vi "Main.vi"() -> ()   [LabVIEW 2024]
doc: "This small application is only a proof of concept. When we have parameters or user data inside an application that could be modified (by the user) at run time, it is important that those changes are 'memorized' when the application is shut down. The next time the application is started it should keep the last configuration made. This is what this application does.\n\nEvery time the user changes the FP data, the changes are saved in the .ini file. If the user closes the application, the FP data is already saved in the .ini configuration file. The next time it is turned on, the data will be loaded again.\n\nIf the user modifies any tag or sector name, or any key name (or its value) in the configuration file (and saves these changes) at run time, the Update button updates this information in the FP of the application, it is the data of the gray fields. This may not be useful in a real application."
uses:
  controls/UI Data.ctl
  dependencies/config data path.ctl
  support/Message Queue/Enqueue Message (Array).vi
  support/Message Queue/Enqueue Message (Single).vi
  <vilib>/Utility/error.llb/Error Cluster From Error Code.vi
  <vilib>/ErrorRing/Error Ring.xnode
  support/Message Queue/Message Queue.lvlib
  support/User Event - Stop/User Event - Stop.lvlib
  dependencies/API Path Config Files Management.lvlib
panel:
  in  "folder path":path
  in  "xml file path":path
  out "Display value":string
  in  "Exit":bool
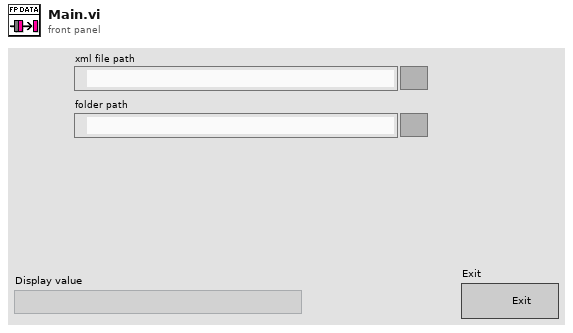
[diagram p1: front panel]
types:
  T1 = typedef "UI Data.ctl" = cluster{"Data Display Ref":refnum<vi>, "Exit Button Ref":refnum<vi>, "xml file Ref":refnum<vi>, "folder path Ref":refnum<vi>, "user path data":T2, "path value idx":i32[]}
  T2 = typedef "API Path Config Files Management.lvlib/config data path.ctl" = cluster{"sections":string[][], "key names":string[], "values":path[]}
  T3 = typedef "NI_LVConfig.lvlib/Config Data RefNum.ctl" = refnum<k1>
  T4 = typedef "Message Queue.lvlib/All Message Queues.ctl" = cluster{"UI":refnum<queue>}
  T5 = enum32{"existing file", "new file", "new or existing file", "existing dir", "new dir", "new or existing dir", "existing file (use LLBs)", "new file (use LLBs)", "new or existing file (use LLBs)", "new or existing file or directory (use LLBs)", "existing dir (use LLBs)", "new dir (use LLBs)", "new or existing dir (use LLBs)", "existing file or dir", "new file or dir", "new or existing file or dir", "existing file or dir (use LLBs)", "new file or dir (use LLBs)"}
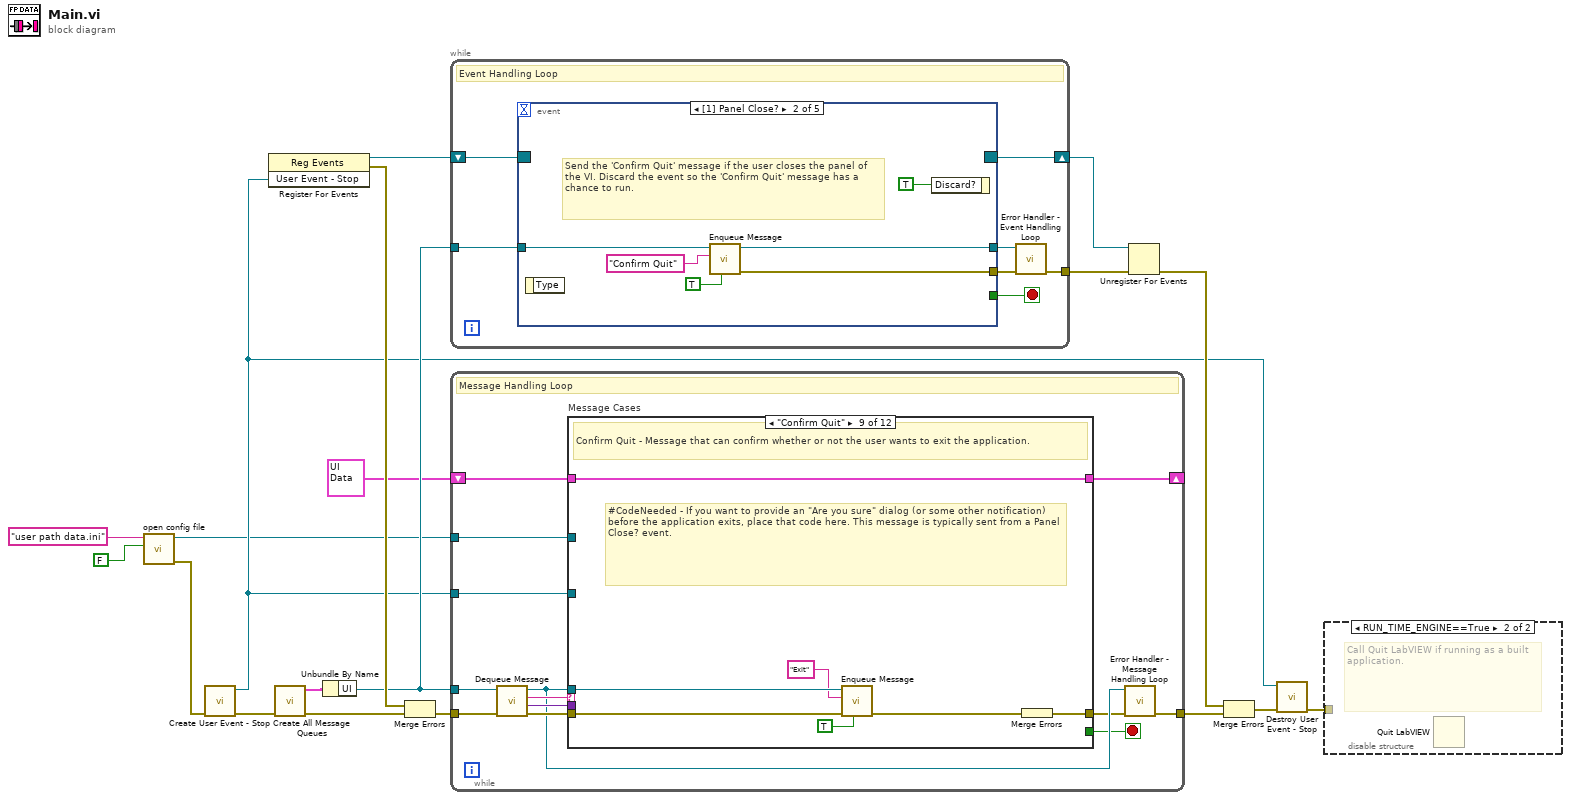
[diagram p0: block diagram]
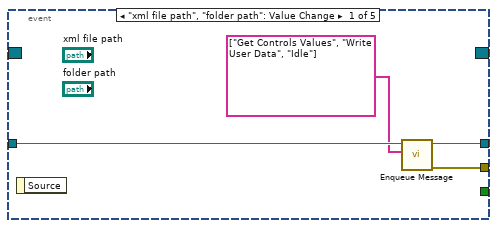
[diagram p3: hidden frame]
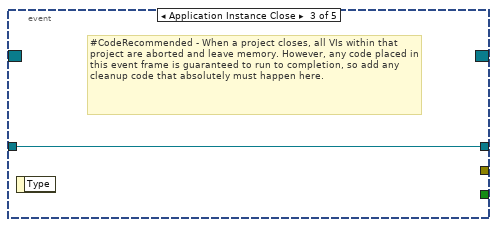
[diagram p4: hidden frame]
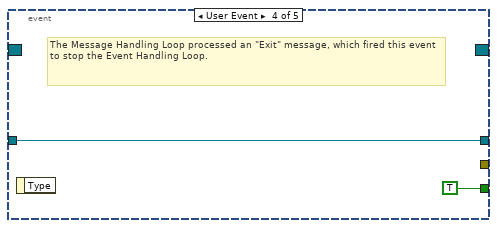
[diagram p5: hidden frame]
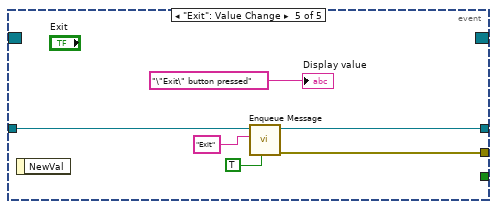
[diagram p6: hidden frame]
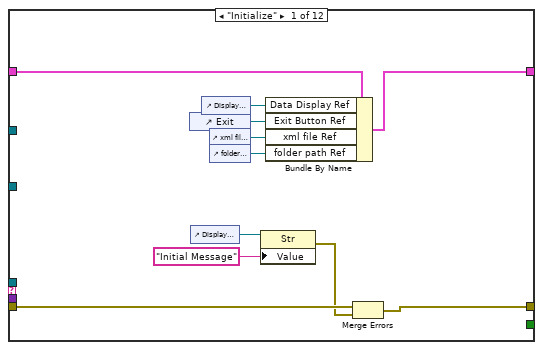
[diagram p7: hidden frame]
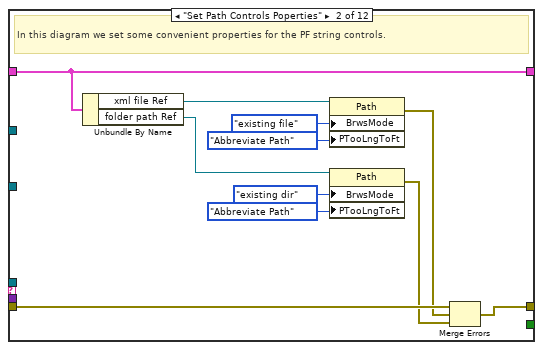
[diagram p8: hidden frame]
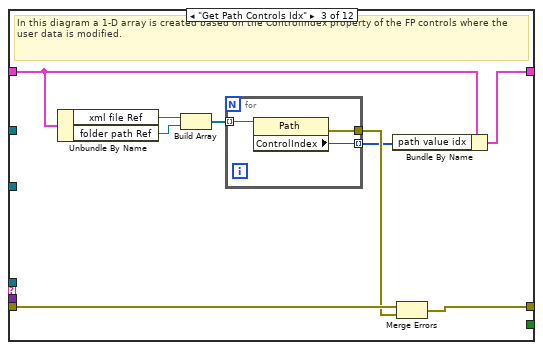
[diagram p9: hidden frame]
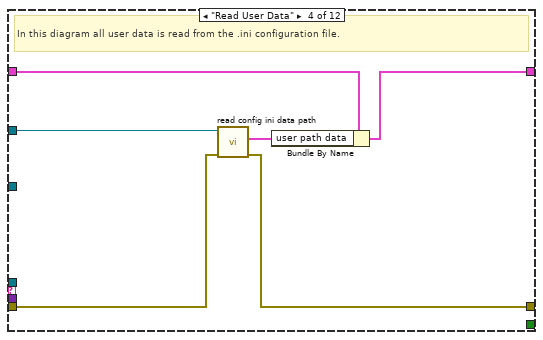
[diagram p10: hidden frame]
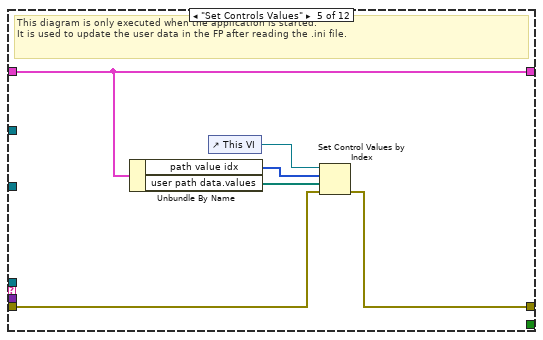
[diagram p11: hidden frame]
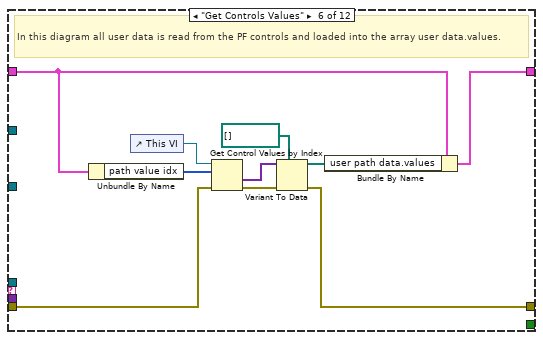
[diagram p12: hidden frame]
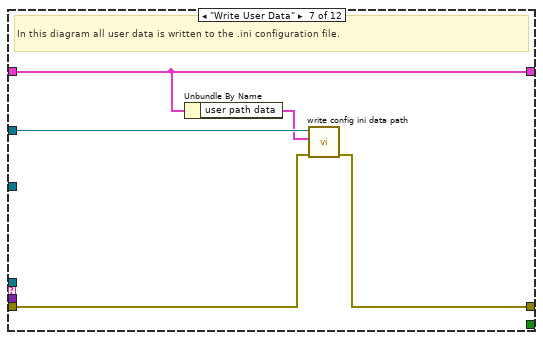
[diagram p13: hidden frame]
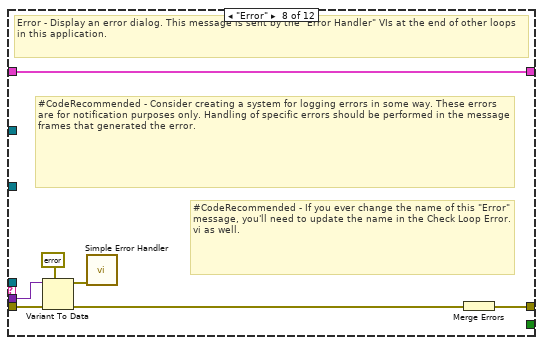
[diagram p14: hidden frame]
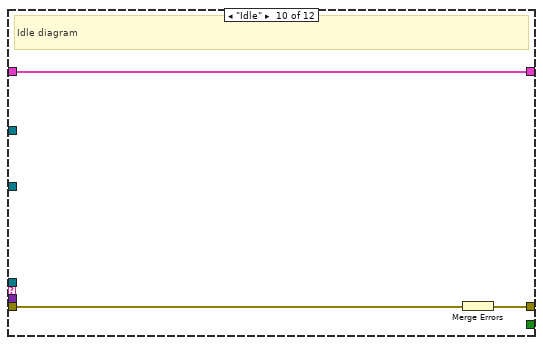
[diagram p15: hidden frame]
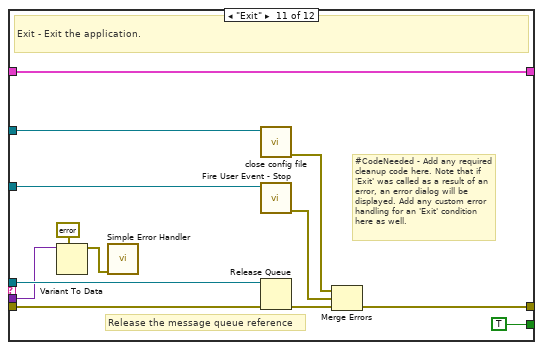
[diagram p16: hidden frame]
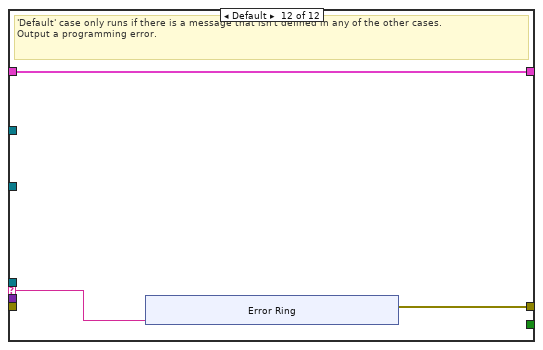
[diagram p17: hidden frame]
diagram:
  n1 = call "open config file.vi"("create file if necessary (T)"=FALSE, "file name"="user path data.ini") -> ("error out"=w2:errorcluster, "Refnum out"=w1:T3)  [unwired: 7 in, 1 out]
  n2 = call "Create User Event - Stop.vi"("error in (no error)"=w2) -> ("error out"=w14:errorcluster, "User Event - Stop"=w5:refnum<user-event>)  [unwired: 9 in]
  n3 = register-events(w5) -> (reference out=w7:refnum<event-registration>, error out=w19:errorcluster)  [unwired: 2 in]
  n4 = call "Create All Message Queues.vi"("error in (no error)"=w14) -> ("error out"=w18:errorcluster, "Message Queues out"=w17:T4)  [unwired: 9 in]
  n5 = Unbundle By Name(w17) -> ("UI"=w15:refnum<queue>)
  n6 = Merge Errors(w19, w18) -> (w6:errorcluster)
  n7 = while {
    tunnel: w15 -> [w26]
    shift-right: [w24] -> w11
    shift-left: w7 -> [w25]
    tunnel: [w20] -> w8
    stop <- w22 stop-if-true
    # "Event Handling Loop"
    n8 = event shown="[1] Panel Close?" {
      selector: w25 -> [_ _ _ _ _]
      dyn-events: [_ _ _ _ _] -> w24
      timeout: _ -> [_ _ _ _ _]
      tunnel: [_ _ _ TRUE ("Discard?") _] -> w22
      tunnel: w26 -> [w30 w35 w37 w39 w45]
      tunnel: [w28 w34 _ _ w44] -> w23
      tunnel: [w29 w33 w37 w39 w43] -> w21
      event "xml file path", "folder path": Value Change {
        n9 = event-data() -> ()  [unwired: 1 in, 1 out]
        n10 = call-poly "Enqueue Message.vi"("Message Array"=string[] ["Get Controls Values", "Write User Data", "Idle"], "Message Queue"=w30) -> ("error out"=w28:errorcluster, "dup Message Queue"=w29:refnum<queue>)  [unwired: 8 in]
      }
      event Panel Close? {
        # "Send the 'Confirm Quit' message if the user closes the panel of the VI. Discard the event so the 'Confirm Quit' message has a chance to run."
        n11 = event-data() -> ()  [unwired: 1 in, 1 out]
        n12 = call-poly "Enqueue Message.vi"("Priority Message? (F)"=TRUE, "Message"="Confirm Quit", "Message Queue"=w35) -> ("error out"=w34:errorcluster, "dup Message Queue"=w33:refnum<queue>)  [unwired: 7 in]
        n13 = event-data("Discard?"=TRUE) -> ()  [unwired: 1 in, 1 out]
      }
      event Application Instance Close {
        # "#CodeRecommended - When a project closes, all VIs within that project are aborted and leave memory. However, any code placed in this event frame is guaranteed to run to completion, so add any cleanup code that absolutely must happen here."
        n14 = event-data() -> ()  [unwired: 1 in, 1 out]
      }
      event User Event {
        # "The Message Handling Loop processed an \"Exit\" message, which fired this event to stop the Event Handling Loop."
        n15 = event-data() -> ()  [unwired: 1 in, 1 out]
      }
      event "Exit": Value Change {
        n16 = event-data() -> ()  [unwired: 1 in, 1 out]
        n17 = call-poly "Enqueue Message.vi"("Priority Message? (F)"=TRUE, "Message"="Exit", "Message Queue"=w45) -> ("error out"=w44:errorcluster, "dup Message Queue"=w43:refnum<queue>)  [unwired: 7 in]
        "Display value" <- "\"Exit\" button pressed" ("Initial Message")
      }
    }
    n18 = call "Error Handler - Event Handling Loop.vi"("error in (no error)"=w23, "Message Queue"=w21) -> ("dup error in"=w20:errorcluster)  [unwired: 8 in, 1 out]
  }
  n19 = while {
    tunnel: w15 -> [w52]
    shift-right: [w48] -> _
    shift-left: T1 {"Data Display Ref"=refnum, "Exit Button Ref"=refnum, "xml file Ref"=refnum, "folder path Ref"=refnum, "user path data"={"sections"=[], "key names"=[], "values"=[]}, "path value idx"=[]} ("Data Cluster") -> [w58]
    tunnel: w5 -> [w57]
    tunnel: w6 -> [w56]
    tunnel: [w50] -> w16
    tunnel: w1 -> [w46]
    stop <- w47 stop-if-true
    # "Message Handling Loop"
    n20 = call "Dequeue Message.vi"("error in (no error)"=w56, "Message Queue"=w52) -> ("error out"=w55:errorcluster, "Message Data"=w53:variant, "Message"=w54:string, "dup Message Queue"=w51:refnum<queue>)  [unwired: 6 in]
    n21 = case "Message Cases" shown="\"Confirm Quit\"" w54 {
      selector: w54 -> [_ _ _ _ _ _ _ _ _ _ _ w150]
      tunnel: w51 -> [_ _ _ _ _ _ _ _ w129 _ w149 _]
      tunnel: w55 -> [w65 w80 w89 w96 w103 w109 w117 w126 w133 w136 w142 _]
      tunnel: [w60 w78 w86 w94 w99 w106 w118 w120 w131 w134 w145 w151] -> w49
      tunnel: w58 -> [w69 w79 w83 w98 w104 w113 w119 w125 w132 w135 w148 w152]
      tunnel: [w68 w79 w88 w97 w104 w114 w119 w125 w132 w135 w148 w152] -> w48
      tunnel: [_ _ _ _ _ _ _ _ _ _ TRUE _] -> w47
      tunnel: w53 -> [_ _ _ _ _ _ _ w124 _ _ w139 _]
      tunnel: w57 -> [_ _ _ _ _ _ _ _ _ _ w144 _]
      tunnel: w46 -> [_ _ _ w93 _ _ w116 _ _ _ w138 _]
      frame "Initialize" {
        n22 = control-ref of="Exit"() -> (w66:refnum<vi>)
        n23 = control-ref of="Display value"() -> (w62:refnum<vi>)
        n24 = control-ref of="Display value"() -> (w67:refnum<vi>)
        n25 = control-ref of="xml file path"() -> (w64:refnum<vi>)
        n26 = control-ref of="folder path"() -> (w63:refnum<vi>)
        n27 = property class="Str"(reference=w62, "Value"="Initial Message" ("Initial Message")) -> (error out=w59:errorcluster)  [unwired: 1 in, 1 out]
        n28 = Bundle By Name(cluster=w69, "Data Display Ref"=w67, "Exit Button Ref"=w66, "xml file Ref"=w64, "folder path Ref"=w63) -> (w68:T1)
        n29 = Merge Errors(w65, w59) -> (w60:errorcluster)
      }
      frame "Set Path Controls Poperties" {
        # "In this diagram we set some convenient properties for the PF string controls."
        n30 = Unbundle By Name(w79) -> ("xml file Ref"=w76:refnum<vi>, "folder path Ref"=w73:refnum<vi>)
        n31 = property class="Path"(reference=w76, "BrwsMode"=T5."existing file" ("Browse Options:Selection Mode"), "PTooLngToFt"=enum32{"Abbreviate Path", "Clip Path"}."Abbreviate Path" ("Path Too Long To Fit")) -> (error out=w77:errorcluster)  [unwired: 1 in, 1 out]
        n32 = property class="Path"(reference=w73, "BrwsMode"=T5."existing dir" ("Browse Options:Selection Mode"), "PTooLngToFt"=enum32{"Abbreviate Path", "Clip Path"}."Abbreviate Path" ("Path Too Long To Fit")) -> (error out=w70:errorcluster)  [unwired: 1 in, 1 out]
        n33 = Merge Errors(w80, w77, w70) -> (w78:errorcluster)
      }
      frame "Get Path Controls Idx" {
        # "In this diagram a 1-D array is created based on the ControlIndex property of the FP controls where the user data is modified."
        n34 = Unbundle By Name(w83) -> ("xml file Ref"=w82:refnum<vi>, "folder path Ref"=w81:refnum<vi>)
        n35 = Build Array(w82, w81) -> (w87:refnum<vi>[])
        n36 = for {
          tunnel: [w92] -> w84 mode=indexing
          tunnel: [w90] -> w85
          tunnel: w87 -> [w91] mode=indexing
          n37 = property class="Path"(reference=w91) -> (error out=w90:errorcluster, "ControlIndex"=w92:i32)  [unwired: 1 in, 1 out]
        }
        n38 = Bundle By Name(cluster=w83, "path value idx"=w84) -> (w88:T1)
        n39 = Merge Errors(w89, w85) -> (w86:errorcluster)
      }
      frame "Read User Data" {
        # "In this diagram all user data is read from the .ini configuration file."
        n40 = call "read config ini data path.vi"("error in (no error)"=w96, "Refnum in"=w93) -> ("error out"=w94:errorcluster, "data out"=w95:T2)  [unwired: 7 in, 1 out]
        n41 = Bundle By Name(cluster=w98, "user path data"=w95) -> (w97:T1)
      }
      frame "Set Controls Values" {
        # "This diagram is only executed when the application is started.\nIt is used to update the user data in the FP after reading the .ini file."
        n42 = Unbundle By Name(w104) -> ("path value idx"=w101:i32[], "user path data.values"=w100:path[])
        n43 = control-ref of="This VI"() -> (w102:refnum<vi>)
        n44 = Set Control Values by Index(0:w102, 1:w101, 2:w100, 3:w103) -> (11:w99:errorcluster)
      }
      frame "Get Controls Values" {
        # "In this diagram all user data is read from the PF controls and loaded into the array user data.values."
        n45 = Unbundle By Name(w113) -> ("path value idx"=w110:i32[])
        n46 = control-ref of="This VI"() -> (w111:refnum<vi>)
        n47 = Get Control Values by Index(0:w111, 1:w110, 3:w109) -> (10:w112:variant[], 11:w107:errorcluster)
        n48 = Variant To Data(error in=w107, type=path[] [] ("user path data.values"), Variant=w112) -> (data=w108:path[], error out=w106:errorcluster)
        n49 = Bundle By Name(cluster=w113, "user path data.values"=w108) -> (w114:T1)
      }
      frame "Write User Data" {
        # "In this diagram all user data is written to the .ini configuration file."
        n50 = Unbundle By Name(w119) -> ("user path data"=w115:T2)
        n51 = call "write config ini data path.vi"("error in (no error)"=w117, "data in"=w115, "Refnum in"=w116) -> ("error out"=w118:errorcluster)  [unwired: 7 in, 1 out]
      }
      frame "Error" {
        # "#CodeRecommended - If you ever change the name of this \"Error\" message, you'll need to update the name in the Check Loop Error.vi as well."
        # "#CodeRecommended - Consider creating a system for logging errors in some way. These errors are for notification purposes only. Handling of specific errors should be performed in the message frames that generated the error."
        # "Error - Display an error dialog. This message is sent by the \"Error Handler\" VIs at the end of other loops in this application."
        n52 = Variant To Data(error in=w126, type=errorcluster {"status"=FALSE, "code"=0, "source"=""} ("error constant"), Variant=w124) -> (data=w122:errorcluster, error out=w121:errorcluster)
        n53 = call <vilib>:"Simple Error Handler.vi"("error in (no error)"=w122) -> ()  [unwired: 4 in, 5 out]
        n54 = Merge Errors(w121) -> (w120:errorcluster)
      }
      frame "Confirm Quit" {
        # "#CodeNeeded - If you want to provide an \"Are you sure\" dialog (or some other notification) before the application exits, place that code here. This message is typically sent from a Panel Close? event."
        # "Confirm Quit - Message that can confirm whether or not the user wants to exit the application."
        n55 = call-poly "Enqueue Message.vi"("Priority Message? (F)"=TRUE, "error in (no error)"=w133, "Message"="Exit", "Message Queue"=w129) -> ("error out"=w130:errorcluster)  [unwired: 6 in, 1 out]
        n56 = Merge Errors(w130) -> (w131:errorcluster)
      }
      frame "Idle" {
        # "Idle diagram"
        n57 = Merge Errors(w136) -> (w134:errorcluster)
      }
      frame "Exit" {
        # "Release the message queue reference"
        # "#CodeNeeded - Add any required cleanup code here. Note that if 'Exit' was called as a result of an error, an error dialog will be displayed. Add any custom error handling for an 'Exit' condition here as well."
        # "Exit - Exit the application."
        n58 = Variant To Data(type=errorcluster {"status"=FALSE, "code"=0, "source"=""} ("error constant"), Variant=w139) -> (data=w140:errorcluster)  [unwired: 1 in, 1 out]
        n59 = call <vilib>:"Simple Error Handler.vi"("error in (no error)"=w140) -> ()  [unwired: 4 in, 5 out]
        n60 = call "close config file.vi"("Refnum in"=w138) -> ("error out"=w137:errorcluster)  [unwired: 10 in]
        n61 = call "Fire User Event - Stop.vi"("User Event - Stop"=w144) -> ("error out"=w143:errorcluster)  [unwired: 10 in]
        n62 = Release Queue(queue=w149, error in (no error)=w142) -> (error out=w146:errorcluster)  [unwired: 1 in, 2 out]
        n63 = Merge Errors(w137, w143, w146) -> (w145:errorcluster)
      }
      frame Default {
        # "'Default' case only runs if there is a message that isn't defined in any of the other cases.\nOutput a programming error."
        n64 = xnode "Error Ring"("parameter 0"=w150) -> ("error out"=w151:errorcluster)
      }
    }
    n65 = call "Error Handler - Message Handling Loop.vi"("error in (no error)"=w49, "Message Queue"=w51) -> ("dup error in"=w50:errorcluster)  [unwired: 8 in, 1 out]
  }
  n66 = Unregister For Events(event registration refnum=w11, error in=w8) -> (error out=w12:errorcluster)
  n67 = Merge Errors(w12, w16) -> (w13:errorcluster)
  n68 = call "Destroy User Event - Stop.vi"("error in (no error)"=w13, "User Event - Stop"=w5) -> ("error out"=w9:errorcluster)  [unwired: 9 in]
  n69 = disable-structure shown="RUN_TIME_ENGINE==True" {
    disable-tunnel: w9 -> [_ _]
    frame condition #0 (active) {
    }
    frame condition #1 {
      # "Call Quit LabVIEW if running as a built application."
      n70 = Quit LabVIEW() -> ()  [unwired: 1 in]
    }
  }
